vi "GEECS IMAQdx set attribute.vi"(8 "error in (no error)":errorcluster, 9 "Attribute value":string, 10 "Attribute name":string, 11 "Refnum in":T1) -> (0 "error out":errorcluster, 3 "Refnum out":T1)   [LabVIEW 2020]
uses:
  <vilib>/userDefined/High Color/IMAQdx.ctl
  <resource>/objmgr/imaqdx.rc
  <vilib>/vision/driver/NI_Vision_Acquisition_Software.lvlib
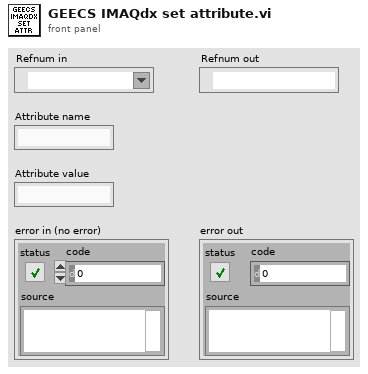
[diagram p1: front panel]
types:
  T1 = typedef "IMAQdx.ctl" = refnum<k21>
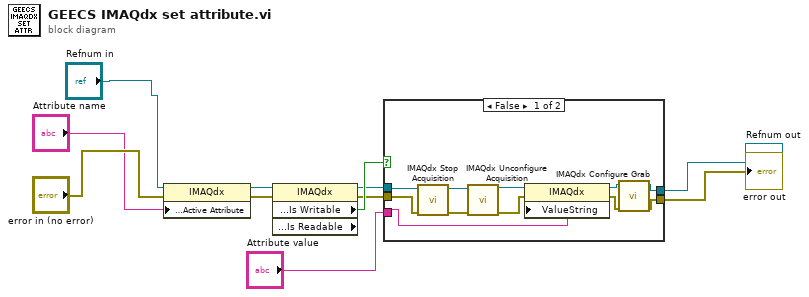
[diagram p0: block diagram]
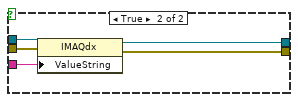
[diagram p2: hidden frame]
diagram:
  n1 = property class="IMAQdx"(reference="Refnum in", error in="error in (no error)", "Camera Attributes:Active Attribute"="Attribute name") -> (reference out=w6:T1, error out=w8:errorcluster)
  n2 = property class="IMAQdx" props=["Camera Attributes:Is Writable", "Camera Attributes:Is Readable"](reference=w6, error in=w8) -> (reference out=w9:T1, error out=w10:errorcluster, "Camera Attributes:Is Writable"=w11:bool)  [unwired: 1 out]
  n3 = case shown="False" w11 {
    tunnel: "Attribute value" -> [w17 w27]
    tunnel: [w14 w26] -> w2
    tunnel: [w13 w25] -> w3
    tunnel: w9 -> [w21 w24]
    tunnel: w10 -> [w12 w23]
    frame False {
      n4 = call <vilib>:"IMAQdx Stop Acquisition.vi"("error in"=w12, "Session In"=w21) -> ("error out"=w22:errorcluster, "Session Out"=w20:T1)  [unwired: 8 out]
      n5 = call <vilib>:"IMAQdx Unconfigure Acquisition.vi"("error in"=w22, "Session In"=w20) -> ("error out"=w18:errorcluster, "Session Out"=w19:T1)  [unwired: 8 out]
      n6 = property class="IMAQdx"(reference=w19, error in=w18, "ValueString"=w17) -> (reference out=w16:T1, error out=w15:errorcluster)
      n7 = call <vilib>:"IMAQdx Configure Grab.vi"("error in"=w15, "Session In"=w16) -> ("error out"=w13:errorcluster, "Session Out"=w14:T1)  [unwired: 1 in, 7 out]
    }
    frame True {
      n8 = property class="IMAQdx"(reference=w24, error in=w23, "ValueString"=w27) -> (reference out=w26:T1, error out=w25:errorcluster)
    }
  }
  "error out" <- w3
  "Refnum out" <- w2
